vi "UnRegisterPubSub.vi"(2 "LogPath in":path, 3 "ROS":T4) -> (0 "LogPath out":path, 1 "MyState":T3)   [LabVIEW 2012]
doc: "Unregisters a publisher or subscriber with the master"
uses:
  <userlib>/ROSforLV/ROS/Code/SubVIs/_ROSControl.ctl
  <userlib>/ROSforLV/ROS/Code/SubVIs/_ROSDirection.ctl
  <userlib>/ROSforLV/ROS/Code/Console/Servers/ServerSubs/MyState.ctl
  <userlib>/ROSforLV/ROS/Code/Console/Servers/ServerSubs/ROSLog.ctl
  <userlib>/ROSforLV/ROS/Code/_ROSDefinition.vi
panel:
  out "unReply":T1
  out "Log":T2
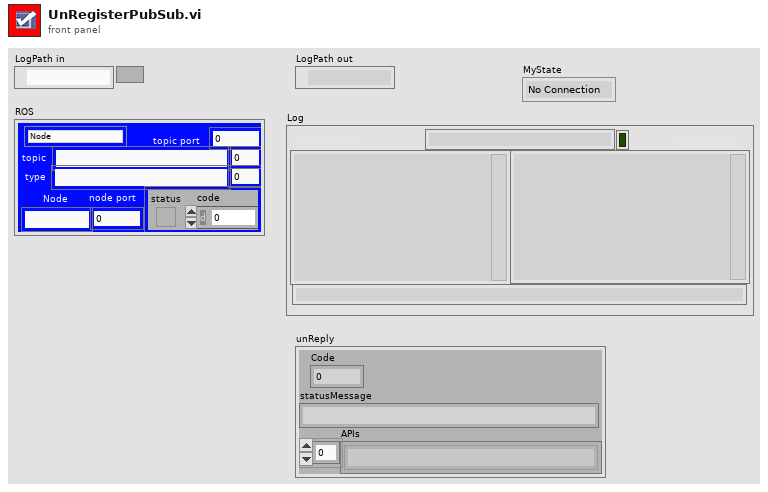
[diagram p1: front panel]
types:
  T1 = cluster{"Code":i8, "statusMessage":string, "APIs":string[]}
  T2 = typedef "ROSLog.ctl" = cluster{"Sent":string, "Reply":string, "MethodName":string, "success":bool, "Dir1":string, "Dir2":string, "Time Stamp":string, "error":errorcluster, "Preamble":string, "Midamble":string, "Postamble":string}
  T3 = typedef "MyState.ctl" = enum16{"No Connection", "Registered", "Connected", "Close"}
  T4 = typedef "_ROSControl.ctl" = cluster{"topic port":u16, "Node":string, "topic":string, "type":string, "node port":u16, "error ":errorcluster, "Direction":T5, "Update (ms)":u16, "FIFO size":u16}
  T5 = typedef "_ROSDirection.ctl" = enum16{"Node", "Publisher", "Subscriber", "ServiceClient", "ServiceProvider"}
  T6 = cluster{"Caller ID":string, "Topic":string, "Caller API":string}
  T7 = enum16{"http://IP:port", "http://IP", "IP:port", "IP only"}
  T8 = cluster{"Code":i8, "statusMessage":string, "APIs":string[]}[]
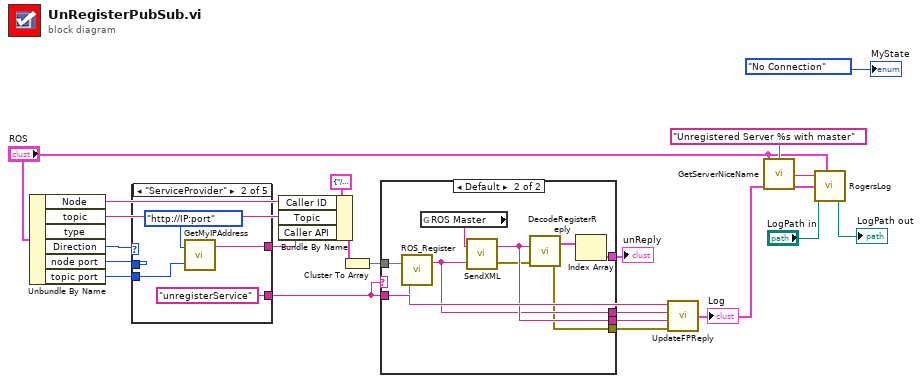
[diagram p0: block diagram]
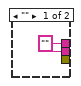
[diagram p2: hidden frame]
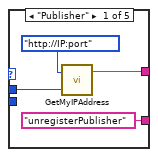
[diagram p3: hidden frame]
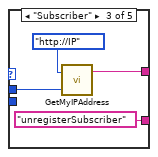
[diagram p4: hidden frame]
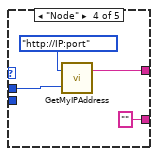
[diagram p5: hidden frame]
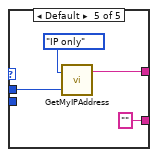
[diagram p6: hidden frame]
diagram:
  n1 = Unbundle By Name("ROS") -> ("Node"=w10:string, "topic"=w9:string, "Direction"=w8:T5, "node port"=w11:u16, "topic port"=w1:u16)  [unwired: 1 out]
  n2 = case shown="\"ServiceProvider\"" w8 {
    tunnel: [w25 w29 w33 w37 w41] -> w7
    tunnel: w11 -> [w23 _ w31 w36 w40]
    tunnel: ["unregisterPublisher" ("Method Name") "unregisterService" ("Method Name") "unregisterSubscriber" ("Method Name") "" ("Method Name") "" ("Method Name")] -> w20
    tunnel: w1 -> [_ w26 _ _ _]
    frame "Publisher" {
      n3 = call <userlib>:"GetMyIPAddress.vi"("Port"=w23, "Format"=T7."http://IP:port") -> ("URI"=w25:string)  [unwired: 1 out]
    }
    frame "ServiceProvider" {
      n4 = call <userlib>:"GetMyIPAddress.vi"("Port"=w26, "Format"=T7."http://IP:port") -> ("URI"=w29:string)  [unwired: 1 out]
    }
    frame "Subscriber" {
      n5 = call <userlib>:"GetMyIPAddress.vi"("Port"=w31, "Format"=T7."http://IP") -> ("URI"=w33:string)  [unwired: 1 out]
    }
    frame "Node" {
      n6 = call <userlib>:"GetMyIPAddress.vi"("Port"=w36, "Format"=T7."http://IP:port") -> ("URI"=w37:string)  [unwired: 1 out]
    }
    frame Default {
      n7 = call <userlib>:"GetMyIPAddress.vi"("Port"=w40, "Format"=T7."IP only") -> ("URI"=w41:string)  [unwired: 1 out]
    }
  }
  n8 = Bundle By Name(cluster=T6 {"Caller ID"="/labview", "Topic"="/topic", "Caller API"="API"} ("Parameters"), "Caller ID"=w10, "Topic"=w9, "Caller API"=w7) -> (w16:T6)
  n9 = Cluster To Array(cluster=w16) -> (array=w15:string[])
  n10 = case shown="Default" w20 {
    tunnel: [w42 w51] -> w13
    tunnel: [w42 w50] -> w14
    tunnel: w15 -> [_ w49]
    tunnel: [_ w45] -> w17
    tunnel: [_ w44] -> w19
    tunnel: w20 -> [_ w43]
    frame "" {
      w42 = "" ("registerSubscriber")
    }
    frame Default {
      n11 = call <userlib>:"ROS_Register.vi"("Parameters"=w49, "Method Name"=w43) -> ("registerSubscriber"=w50:string)  [unwired: 1 in]
      n12 = global read "_ROSDefinition.vi" "ROS Master"() -> (w46:string)
      n13 = call <userlib>:"SendXML.vi"("Send"=w50, "URI in"=w46) -> ("error out"=w48:errorcluster, "Reply"=w51:string)
      n14 = call <userlib>:"DecodeRegisterReply.vi"("error in (no error)"=w48, "Response"=w51) -> ("error out"=w45:errorcluster, "Reply"=w47:T8)
      n15 = Index Array(array=w47) -> (element=w44:T1)  [unwired: 1 in]
    }
  }
  "unReply" <- w19
  n16 = call <userlib>:"UpdateFPReply.vi"("error in (no error)"=w17, "Reply"=w13, "Sent"=w14, "method"=w20) -> ("Log"=w18:T2)
  "Log" <- w18
  n17 = call <userlib>:"GetServerNiceName.vi"("ROS"="ROS", "Text to add"="Unregistered Server %s with master") -> ("String"=w12:string)
  n18 = call <userlib>:"RogersLog.vi"("Text to add"=w12, "ROS"="ROS", "Log"=w18, "LogPath in"="LogPath in") -> ("LogPath out"=→"LogPath out":path)  [unwired: 1 in, 1 out]
  "MyState" <- MyState."No Connection" ("MyState")
